vi "RETURN PGSQL ITEMS.vi"(11 "REFERENCES":T1) -> ()   [LabVIEW 2019]
uses:
  Controls/References Cluster.ctl
  Controls/Custom Calendar/Custom Calendar.xctl
  Controls/Table Data Types/Inventory Data Type.ctl
  Controls/Table Data Types/Checked In Archive Data Type.ctl
  <vilib>/addons/database/Connection.llb/DB Tools Open Connec (String).vi
  <vilib>/addons/database/Connection.llb/Conn Execute.vi
  <vilib>/addons/database/Recordset.llb/Rec Fetch Recordset Data (R).vi
  <vilib>/addons/database/Recordset.llb/Rec Destroy - Connection.vi
  <vilib>/addons/database/_DB Variant To Data/Database Variant To Data.xnode
  <vilib>/addons/database/NI_Database_API.lvlib
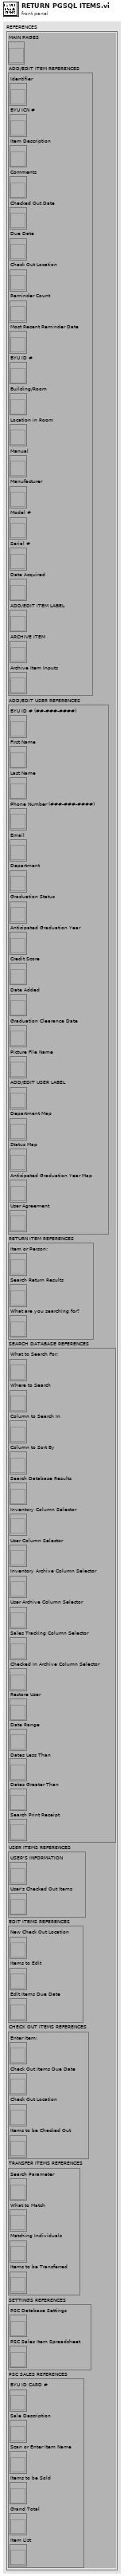
[diagram p1: front panel]
types:
  T1 = typedef "References Cluster.ctl" = cluster{"MAIN PAGES":refnum<vi>, "ADD/EDIT ITEM REFERENCES":cluster{"Identifier":refnum<vi>, "BYU ICN #":refnum<vi>, "Item Description":refnum<vi>, "Comments":refnum<vi>, "Checked Out Date":refnum<vi>, "Due Date":refnum<vi>, "Check Out Location":refnum<vi>, "Reminder Count":refnum<vi>, "Most Recent Reminder Date":refnum<vi>, "BYU ID #":refnum<vi>, "Building/Room":refnum<vi>, "Location in Room":refnum<vi>, "Manual":refnum<vi>, "Manufacturer":refnum<vi>, "Model #":refnum<vi>, "Serial #":refnum<vi>, "Date Acquired":refnum<vi>, "ADD/EDIT ITEM LABEL":refnum<vi>, "ARCHIVE ITEM":refnum<vi>, "Archive Item Inputs":refnum<vi>}, "ADD/EDIT USER REFERENCES":cluster{"BYU ID # (##-###-####)":refnum<vi>, "First Name":refnum<vi>, "Last Name":refnum<vi>, "Phone Number (###-###-####)":refnum<vi>, "Email":refnum<vi>, "Department":refnum<vi>, "Graduation Status":refnum<vi>, "Anticipated Graduation Year":refnum<vi>, "Credit Score":refnum<vi>, "Date Added":refnum<vi>, "Graduation Clearance Date":refnum<vi>, "Picture File Name":refnum<vi>, "ADD/EDIT USER LABEL":refnum<vi>, "Department Map":refnum<vi>, "Status Map":refnum<vi>, "Anticipated Graduation Year Map":refnum<vi>, "User Agreement":refnum<vi>}, "RETURN ITEM REFERENCES":cluster{"Item or Person:":refnum<vi>, "Search Return Results":refnum<vi>, "What are you searching for?":refnum<vi>}, "SEARCH DATABASE REFERENCES":cluster{"What to Search For:":refnum<vi>, "Where to Search":refnum<vi>, "Column to Search In":refnum<vi>, "Column to Sort By":refnum<vi>, "Search Database Results":refnum<vi>, "Inventory Column Selector":refnum<vi>, "User Column Selector":refnum<vi>, "Inventory Archive Column Selector":refnum<vi>, "User Archive Column Selector":refnum<vi>, "Sales Tracking Column Selector":refnum<vi>, "Checked In Archive Column Selector":refnum<vi>, "Restore User":refnum<vi>, "Date Range":refnum<vi>, "Dates Less Than":refnum<vi>, "Dates Greater Than":refnum<vi>, "Search Print Receipt":refnum<vi>}, "USER ITEMS REFERENCES":cluster{"USER'S INFORMATION":refnum<vi>, "User's Checked Out Items":refnum<vi>}, "EDIT ITEMS REFERENCES":cluster{"New Check Out Location":refnum<vi>, "Items to Edit":refnum<vi>, "Edit Items Due Date":refnum<vi>}, "CHECK OUT ITEMS REFERENCES":cluster{"Enter Item:":refnum<vi>, "Check Out Items Due Date":refnum<vi>, "Check Out Location":refnum<vi>, "Items to be Checked Out":refnum<vi>}, "TRANSFER ITEMS REFERENCES":cluster{"Search Parameter":refnum<vi>, "What to Match":refnum<vi>, "Matching Individuals":refnum<vi>, "Items to be Transferred":refnum<vi>}, "SETTINGS REFERENCES":cluster{"PSC Database Settings":refnum<vi>, "PSC Sales Item Spreadsheet":refnum<vi>}, "PSC SALES REFERENCES":cluster{"BYU ID CARD #":refnum<vi>, "Sale Description":refnum<vi>, "Scan or Enter Item Name":refnum<vi>, "Items to be Sold":refnum<vi>, "Grand Total":refnum<vi>, "Item List":refnum<vi>}}
  T2 = cluster{"Item or Person:":refnum<vi>, "Search Return Results":refnum<vi>, "What are you searching for?":refnum<vi>}
  T3 = typedef "NI_Database_API.lvlib/Conn ObjectReference.ctl" = refnum<k1>
  T4 = typedef "Checked In Archive Data Type.ctl" = cluster{"Identifier":string, "BYU ICN #":string, "Item Description":string, "Comments":string, "Checked Out Date":string, "Due Date":string, "Check Out Location":string, "Reminder Count":i32, "Most Recent Reminder Date":string, "BYU ID #":string, "Building/Room":string, "Location in Room":string, "Manual":string, "Manufacturer":string, "Model #":string, "Serial #":string, "Date Acquired":string, "Date Returned":string}
  T5 = typedef "Inventory Data Type.ctl" = cluster{"Identifier":string, "BYU ICN #":string, "Item Description":string, "Comments":string, "Checked Out Date":string, "Due Date":string, "Check Out Location":string, "Reminder Count":i32, "Most Recent Reminder Date":string, "BYU ID #":string, "Building/Room":string, "Location in Room":string, "Manual":string, "Manufacturer":string, "Model #":string, "Serial #":string, "Date Acquired":string}
  T6 = typedef "NI_Database_API.lvlib/Rec ObjectReference.ctl" = refnum<k1>
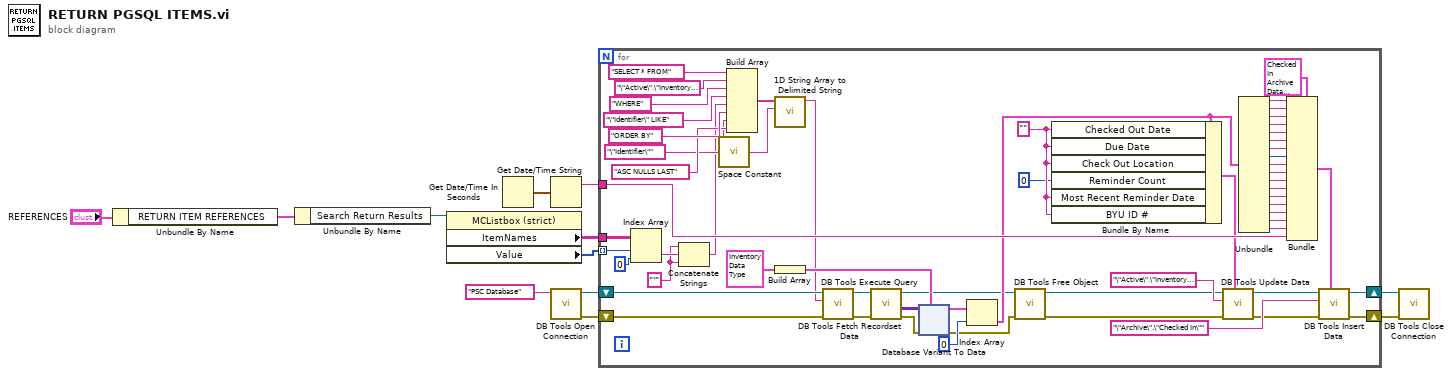
[diagram p0: block diagram]
diagram:
  n1 = Unbundle By Name("REFERENCES") -> ("RETURN ITEM REFERENCES"=w2:T2)
  n2 = Unbundle By Name(w2) -> ("Search Return Results"=w12:refnum<vi>)
  n3 = property class="MCListbox (strict)"(reference=w12) -> ("ItemNames"=w11:string[][], "Value"=w1:i32[])  [unwired: 1 in, 2 out]
  n4 = Get Date/Time In Seconds() -> (seconds since 1Jan1904=w7:timestamp)
  n5 = Get Date/Time String(seconds (now)=w7) -> (date string=w6:string)  [unwired: 2 in, 1 out]
  n6 = call-poly <vilib>:"DB Tools Open Connection.vi"("connection information"="PSC Database") -> ("error out"=w9:errorcluster, "connection reference"=w10:T3)  [unwired: 7 in]
  n7 = for {
    tunnel: w1 -> [w71] mode=indexing
    tunnel: w11 -> [w72]
    shift-right: [w66] -> w5
    shift-left: w10 -> [w36]
    shift-right: [w65] -> w4
    shift-left: w9 -> [w35]
    tunnel: w6 -> [w67]
    w14 = "'" ("string")
    w45 = "" ("Checked Out Date")
    n8 = Index Array(array=w72, index (row)=w71, index (col)=0 ("disabled index (col)")) -> (element=w15:string)
    n9 = Concatenate Strings(w14, w15, w14) -> (w13:string)
    n10 = call <vilib>:"Space Constant.vi"() -> ("String"=w34:string)
    n11 = Build Array("SELECT * FROM" ("SQL query"), "\"Active\".\"Inventory\"", "WHERE", "\"Identifier\" LIKE" ("string"), w13, "ORDER BY" ("string"), "\"Identifier\"" ("string"), "ASC NULLS LAST") -> (w33:string[])
    n12 = call <vilib>:"1D String Array to Delimited String.vi"("delimiter"=w34, "string array"=w33) -> ("delimited string"=w25:string)  [unwired: 9 in]
    n13 = Build Array(T5 {"Identifier"="", "BYU ICN #"="", "Item Description"="", "Comments"="", "Checked Out Date"="", "Due Date"="", "Check Out Location"="", "Reminder Count"=0, "Most Recent Reminder Date"="", "BYU ID #"="", "Building/Room"="", "Location in Room"="", "Manual"="", "Manufacturer"="", "Model #"="", "Serial #"="", "Date Acquired"=""} ("Array")) -> (w63:T5[])
    n14 = call-poly <vilib>:"DB Tools Execute Query.vi"("error in (no error)"=w35, "SQL query"=w25, "connection reference"=w36) -> ("error out"=w24:errorcluster, "recordset reference"=w23:T6)  [unwired: 5 in]
    n15 = call-poly <vilib>:"DB Tools Fetch Recordset Data.vi"("error in (no error)"=w24, "recordset reference"=w23) -> ("error out"=w21:errorcluster, "recordset data"=w22:variant[][], "recordset reference out"=w19:T6)  [unwired: 3 in]
    n16 = xnode "Database Variant To Data"("database variant"=w22, "error in (no error)"=w21, "type"=w63) -> ("data"=w69:T5[], "error out"=w20:errorcluster)
    n17 = Index Array(array=w69, index=0) -> (element=w46:T5)
    n18 = call-poly <vilib>:"DB Tools Free Object.vi"("error in (no error)"=w20, "recordset reference"=w19) -> ("error out"=w17:errorcluster, "connection reference"=w18:T3)  [unwired: 8 in]
    n19 = Bundle By Name(cluster=w46, "Checked Out Date"=w45, "Due Date"=w45, "Check Out Location"=w45, "Reminder Count"=0, "Most Recent Reminder Date"=w45, "BYU ID #"=w45) -> (w44:T5)
    n20 = call <vilib>:"DB Tools Update Data.vi"("data"=w44, "error in (no error)"=w17, "table"="\"Active\".\"Inventory\"", "connection reference"=w18) -> ("error out"=w58:errorcluster, "connection reference out"=w59:T3)  [unwired: 6 in]
    n21 = Unbundle(w46) -> ("Identifier"=w56:string, "BYU ICN #"=w55:string, "Item Description"=w54:string, "Comments"=w53:string, "Checked Out Date"=w52:string, "Due Date"=w51:string, "Check Out Location"=w50:string, "Reminder Count"=w49:i32, "Most Recent Reminder Date"=w48:string, "BYU ID #"=w47:string, "Building/Room"=w37:string, "Location in Room"=w38:string, "Manual"=w39:string, "Manufacturer"=w40:string, "Model #"=w41:string, "Serial #"=w42:string, "Date Acquired"=w43:string)
    n22 = Bundle(cluster=T4 {"Identifier"="", "BYU ICN #"="", "Item Description"="", "Comments"="", "Checked Out Date"="", "Due Date"="", "Check Out Location"="", "Reminder Count"=0, "Most Recent Reminder Date"="", "BYU ID #"="", "Building/Room"="", "Location in Room"="", "Manual"="", "Manufacturer"="", "Model #"="", "Serial #"="", "Date Acquired"="", "Date Returned"=""} ("CHECKED IN ARCHIVE DATA TYPE"), "Identifier"=w56, "BYU ICN #"=w55, "Item Description"=w54, "Comments"=w53, "Checked Out Date"=w52, "Due Date"=w51, "Check Out Location"=w50, "Reminder Count"=w49, "Most Recent Reminder Date"=w48, "BYU ID #"=w47, "Building/Room"=w37, "Location in Room"=w38, "Manual"=w39, "Manufacturer"=w40, "Model #"=w41, "Serial #"=w42, "Date Acquired"=w43, "Date Returned"=w67) -> (w61:T4)
    n23 = call <vilib>:"DB Tools Insert Data.vi"("data"=w61, "error in (no error)"=w58, "table"="\"Archive\".\"Checked In\"", "connection reference"=w59) -> ("error out"=w65:errorcluster, "connection reference out"=w66:T3)  [unwired: 6 in]
  }
  n24 = call <vilib>:"DB Tools Close Connection.vi"("error in (no error)"=w4, "connection reference"=w5) -> ()  [unwired: 5 in, 1 out]
